vi "automatic temperature control.vi"(0 "Control Parameters":T1={"Setpoint"=50.0, "Control bandwidth"=4.0, "Settle bandwidth"=1.0, "Integral time"=30.0, "Int\non"=TRUE, "Derivative time"=0.5, "Der\non"=TRUE, "Settle time"=60.0} {"Settle time" format="%.2f"; "Derivative time" format="%.2f"; "Integral time" format="%.2f"; "Settle bandwidth" format="%.2f"; "Control bandwidth" format="%.2f"; "Setpoint" format="%.2f"}, 11 "error in":errorcluster, 12 "Manual Override":bool, 13 "Normalized Power In (0-1)":dbl format="%.2f", 14 "index (0=init)":i32) -> (2 "settled":bool, 3 "time in settle band":dbl format="%.2f", 4 "power meas (0-1)":dbl format="%.2f", 8 "temp meas":dbl=26.795989484821064 format="%.2f", 15 "error out":errorcluster)   [LabVIEW 2014]
doc: "This vi manages the temperature measurement and power control using a PID algorithm\n\nMatt Strader\nPaul K Dixon\nPhysics 350\nPaul K Dixon"
uses:
  typedefs/control parameters.ctl
panel:
  # "Automatic Temperature Control"
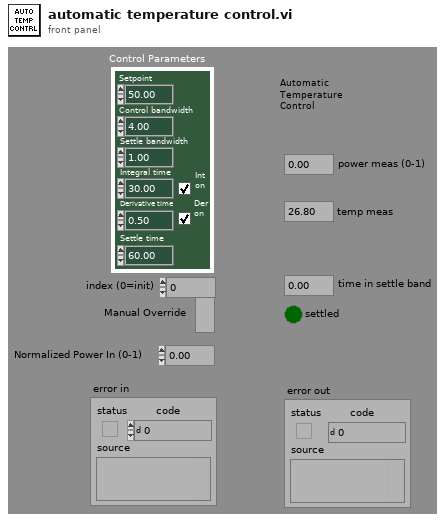
[diagram p1: front panel]
types:
  T1 = typedef "control parameters.ctl" = cluster{"Setpoint":dbl, "Control bandwidth":dbl, "Settle bandwidth":dbl, "Integral time":dbl, "Int\non":bool, "Derivative time":dbl, "Der\non":bool, "Settle time":dbl}
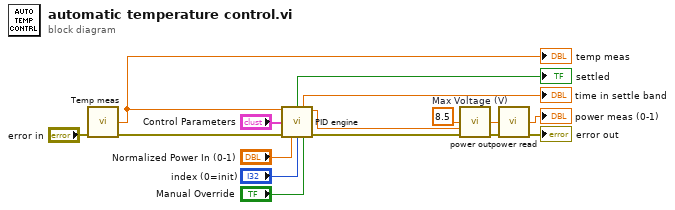
[diagram p0: block diagram]
diagram:
  w1 = 8.5  # Max Voltage (V)
  n1 = call "Temp meas.vi"("error in"="error in") -> ("Temp (deg C)"=w8:dbl, "error out"=w9:errorcluster)  [unwired: 11 in, 2 out]
  "temp meas" <- w8
  n2 = call "PID engine.vi"("Temp In (deg C)"=w8, "Control Parameters"="Control Parameters", "error in"=w9, "Normalized Power In (0-1)"="Normalized Power In (0-1)", "index (0=init)"="index (0=init)", "Manual Override"="Manual Override") -> ("settled"=→"settled":bool, "time in settle band"=→"time in settle band":dbl, "Normalized Power Out (0-1)"=w7:dbl, "error out"=w10:errorcluster)  [unwired: 1 in, 5 out]
  n3 = call "power out.vi"("Max Voltage in (V)"=w1, "Normalized Power (0-1)"=w7, "error in (no error)"=w10) -> ("Max Voltage out (V)"=w14:dbl, "error out"=w13:errorcluster)  [unwired: 11 out]
  n4 = call "power read.vi"("Max Voltage"=w14, "error in (no error)"=w13) -> ("normalized Power Read (0-1)"=→"power meas (0-1)":dbl, "error out"=→"error out":errorcluster)  [unwired: 1 in, 11 out]
